vi "Device Under Test Tester.vi"() -> ()   [LabVIEW 2020]
uses:
  <vilib>/Utility/miscctls.llb/LVStringsAndValuesArrayTypeDef_I32.ctl
  <vilib>/Astemes/Triarc Framework/Application/Application.lvclass
  C:/Program Files (x86)/National Instruments/LabVIEW 2020/vi.lib/Astemes/Triarc Framework/Process/Process.lvclass
  Device Under Test/Device Under Test.lvclass
  <vilib>/Astemes/Triarc Framework/View/View.lvclass
  <vilib>/Astemes/Triarc Framework/Process/Process.lvclass/Process.ctl
  <vilib>/Astemes/Triarc Framework/Process/Private/SubVIs/Wait for finish.vi
  <vilib>/Astemes/Triarc Framework/Process/Private/SubVIs/Set Lifecycle State.vi
  <vilib>/Astemes/Triarc Framework/Process/Protected/Messaging/Send Message.vi
  <vilib>/Astemes/Triarc Framework/Process/Private/SubVIs/Handle Debug Data.vi
  <vilib>/Astemes/Triarc Framework/Process/Public/Lifecycle/Get Lifecycle State.vi
  <vilib>/Utility/error.llb/Error Cluster From Error Code.vi
  <vilib>/Astemes/Triarc Framework/Callback/Callback.lvclass
  <vilib>/Astemes/Triarc Framework/Process/Process.lvclass
panel:
  out "timed out?":bool
  in  "Update DUT Status":bool
  out "Self Test Result":bool
  out "Power State":bool
  in  "Self Test":bool
  in  "Power Off":bool
  in  "Power On":bool
  in  "Refresh Modules":bool
  out "Active Modules":string[](array[string])
  in  "Stop Module":bool
  in  "Select Module":i32(ring)=-1 caption="Select Module\nTo send Request to" items=["All"=-1, "DUT 0"=0]
  in  "Run New Module":bool
  in  "Hide Module Panel":bool
  in  "Show Module Panel":bool
  out "Status":string
  # "This VI tests the API for the Module."
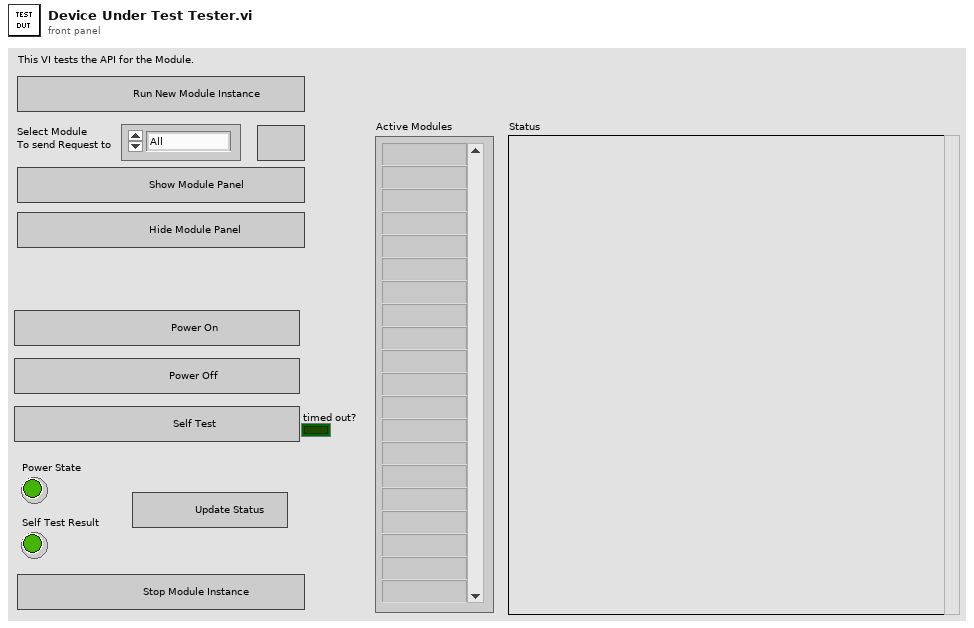
[diagram p1: front panel]
types:
  T1 = typedef "LVStringsAndValuesArrayTypeDef_I32.ctl" = cluster{"String":string, "Value":i32}[]
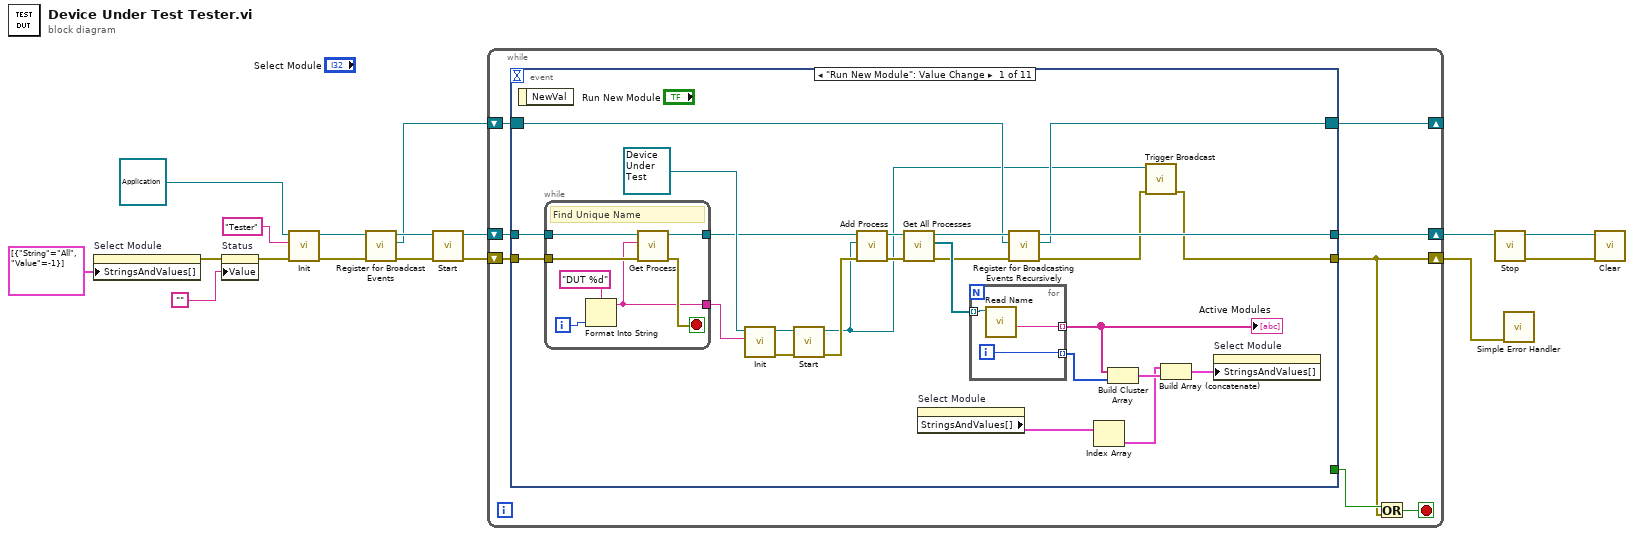
[diagram p0: block diagram]
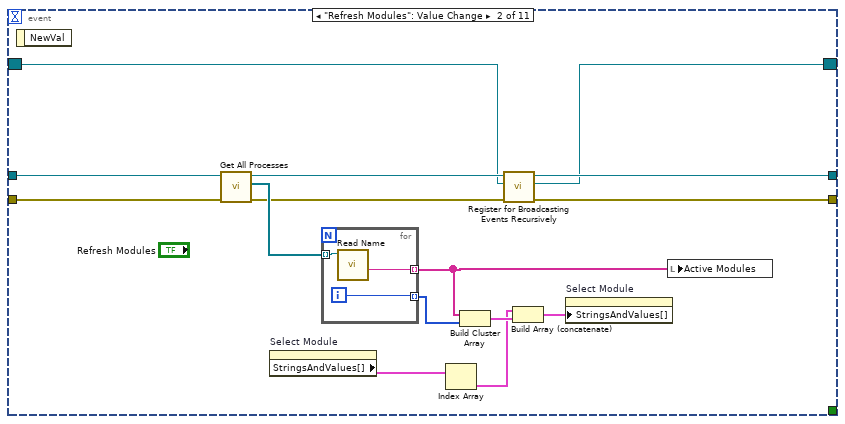
[diagram p2: hidden frame]
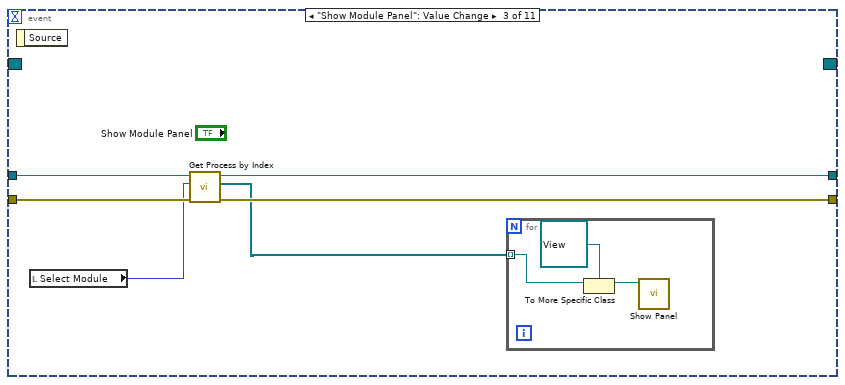
[diagram p3: hidden frame]
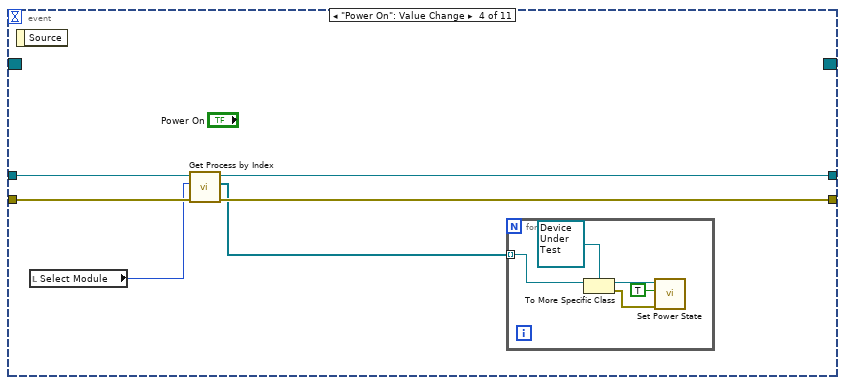
[diagram p4: hidden frame]
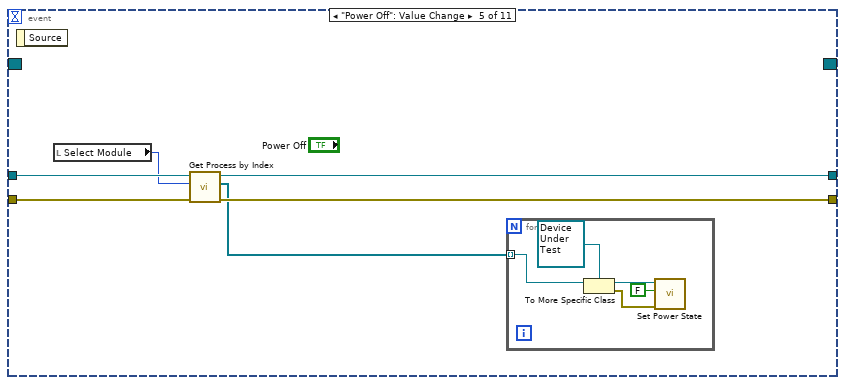
[diagram p5: hidden frame]
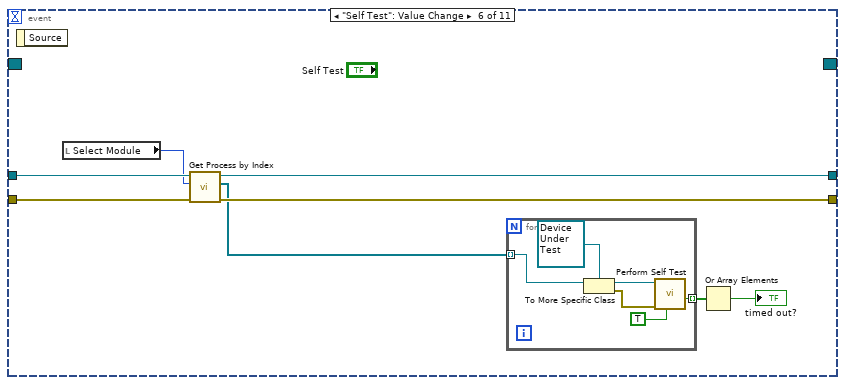
[diagram p6: hidden frame]
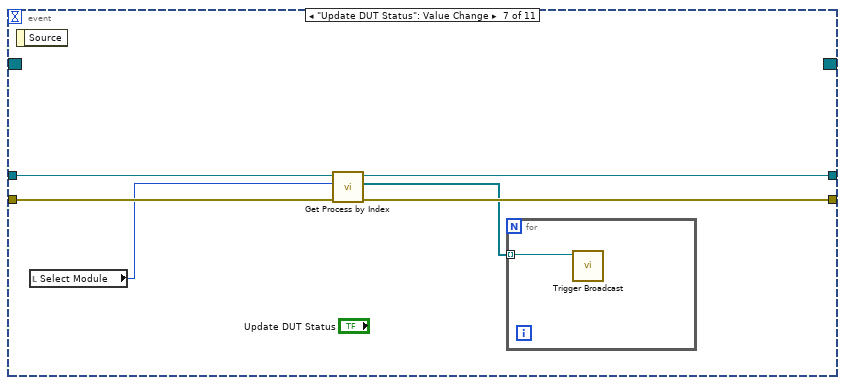
[diagram p7: hidden frame]
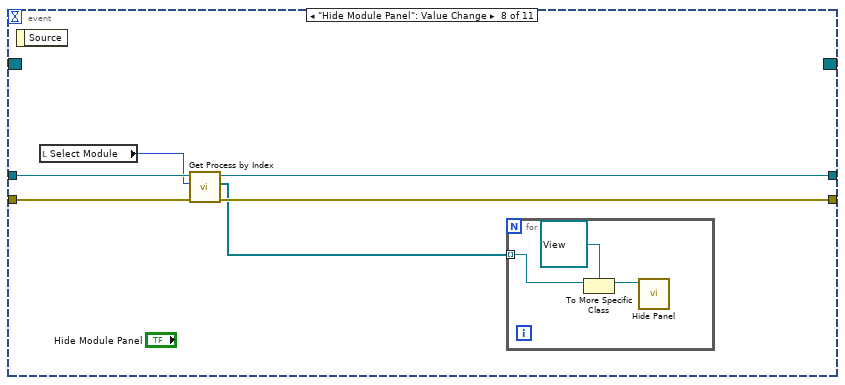
[diagram p8: hidden frame]
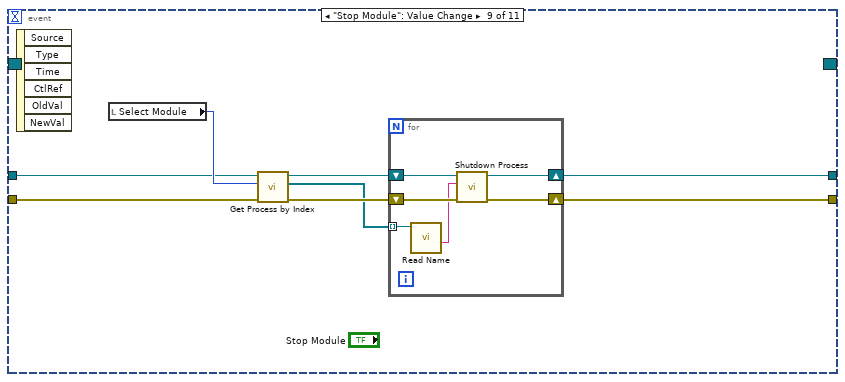
[diagram p9: hidden frame]
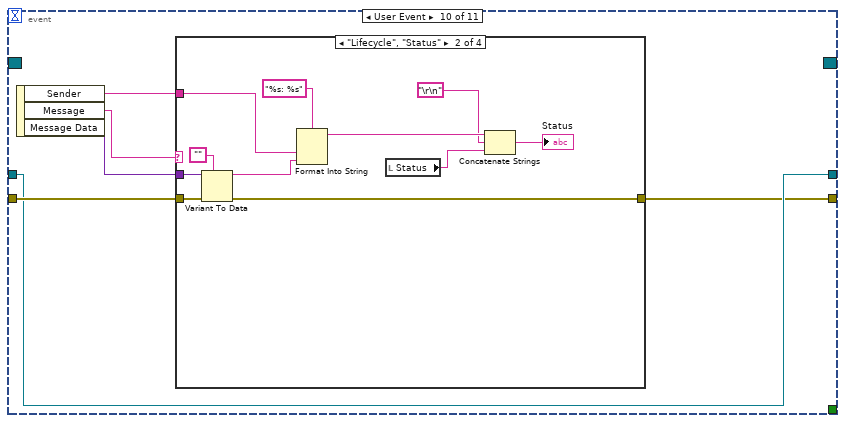
[diagram p10: hidden frame]
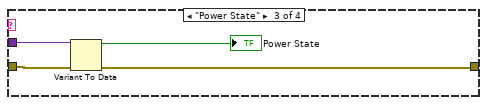
[diagram p12: hidden frame]
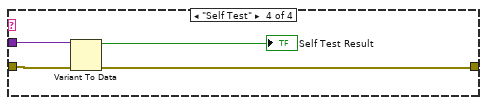
[diagram p13: hidden frame]
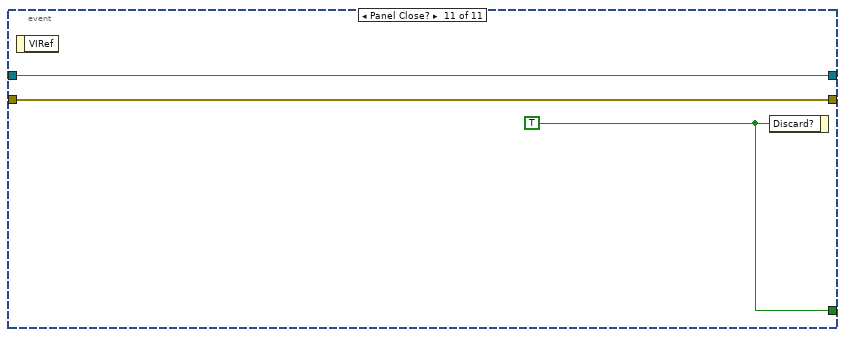
[diagram p14: hidden frame]
diagram:
  n1 = property on="Select Module" class="Ring (strict)"("StringsAndValues[]"=T1 [{"String"="All", "Value"=-1}] ("Strings And Values []")) -> (error out=w3:errorcluster)  [unwired: 2 in, 1 out]
  n2 = property on="Status" class="Str"(error in=w3, "Value"="") -> (error out=w2:errorcluster)  [unwired: 1 in, 1 out]
  n3 = call-dynamic "Init.vi"("error in (no error)"=w2, "Name"="Tester", "Process In"=refnum<class "Application.lvclass"> refnum ("TF.lvlib:Application.lvclass")) -> ("error out"=w4:errorcluster, "Process Out"=w8:refnum<class "Application.lvclass">)  [unwired: 7 in]
  n4 = call <vilib>:"Register for Broadcast Events.vi"("error in (no error)"=w4, "Process In"=w8) -> ("error out"=w6:errorcluster, "Event Registration Refnum Out"=w5:refnum<event-registration>, "Process Out"=w7:refnum<class "Application.lvclass">)  [unwired: 7 in]
  n5 = call <vilib>:"Start.vi"("error in (no error)"=w6, "Process In"=w7) -> ("error out"=w13:errorcluster, "Process Out"=w11:refnum<class "Application.lvclass">)  [unwired: 7 in, 1 out]
  n6 = while {
    shift-right: [w22] -> w17
    shift-left: w13 -> [w25]
    shift-right: [w20] -> w16
    shift-left: w11 -> [w21]
    shift-right: [w18] -> _
    shift-left: w5 -> [w19]
    stop <- w23 stop-if-true
    n7 = event shown="[0] \"Run New Module\": Value Change" {
      selector: w19 -> [w35 w61 _ _ _ _ _ _ _ _ _]
      dyn-events: [w36 w62 _ _ _ _ _ _ _ _ _] -> w18
      timeout: _ -> [_ _ _ _ _ _ _ _ _ _ _]
      tunnel: w25 -> [w32 w70 w84 w93 w104 w117 w129 w136 w145 w158 w181]
      tunnel: [w33 w64 w83 w92 w103 w116 w128 w135 w141 w154 w181] -> w22
      tunnel: [_ _ _ _ _ _ _ _ _ _ w182] -> w24
      tunnel: w21 -> [w31 w69 w82 w91 w102 w115 w127 w134 w146 w156 w180]
      tunnel: [w38 w65 w81 w90 w101 w114 w126 w133 w142 w156 w180] -> w20
      event "Run New Module": Value Change {
        n8 = event-data() -> ()  [unwired: 1 in, 1 out]
        n9 = while {
          tunnel: w32 -> [w56]
          tunnel: w31 -> [w55]
          tunnel: [w54] -> w30
          tunnel: [w51] -> w29
          i -> [w53]
          stop <- w52 stop-if-true
          # "Find Unique Name"
          n10 = Format Into String(format string="DUT %d", w53) -> (resulting string=w51:string)  [unwired: 2 in, 1 out]
          n11 = call <vilib>:"Get Process.vi"("error in (no error)"=w56, "Process Name"=w51, "Application In"=w55) -> ("error out"=w52:errorcluster, "Application Out"=w54:refnum<class "Application.lvclass">)  [unwired: 6 in, 1 out]
        }
        n12 = call-dynamic "Init.vi"("Name"=w29, "View In"=refnum<class "Device Under Test.lvclass"> refnum ("Device Under Test.lvclass")) -> ("error out"=w43:errorcluster, "View Out"=w27:refnum<class "Device Under Test.lvclass">)  [unwired: 8 in]
        n13 = call <vilib>:"Start.vi"("error in (no error)"=w43, "Process In"=w27) -> ("error out"=w28:errorcluster, "Process Out"=w26:refnum<class "Device Under Test.lvclass">)  [unwired: 7 in, 1 out]
        n14 = call <vilib>:"Add Process.vi"("error in (no error)"=w28, "Process"=w26, "Application In"=w30) -> ("error out"=w41:errorcluster, "Application Out"=w42:refnum<class "Application.lvclass">)  [unwired: 7 in]
        n15 = call <vilib>:"Get All Processes.vi"("error in (no error)"=w41, "Application In"=w42) -> ("error out"=w37:errorcluster, "App Processes"=w40:refnum<class "Process.lvclass">[], "Application Out"=w39:refnum<class "Application.lvclass">)  [unwired: 7 in]
        n16 = property on="Select Module" class="Ring (strict)"() -> ("StringsAndValues[]"=w46:T1)  [unwired: 2 in, 2 out]
        n17 = for {
          tunnel: [w58] -> w49 mode=indexing
          tunnel: [w60] -> w48 mode=indexing
          tunnel: w40 -> [w59] mode=indexing
          i -> [w60]
          n18 = call <vilib>:"Read Name.vi"("Process In"=w59) -> ("Name"=w58:string)  [unwired: 7 in, 3 out]
        }
        "Active Modules" <- w49
        n19 = call <vilib>:"Register for Broadcasting Events Recursively.vi"("error in (no error)"=w37, "Event Registration Refnum In"=w35, "Application In"=w39) -> ("error out"=w34:errorcluster, "Event Registration Refnum Out"=w36:refnum<event-registration>, "Application Out"=w38:refnum<class "Application.lvclass">)  [unwired: 6 in]
        n20 = Index Array(array=w46) -> (element=w44:cluster{"String":string, "Value":i32})  [unwired: 1 in]
        n21 = Build Cluster Array(w49, w48) -> (w47:cluster{"Name":string, i32}[])
        n22 = call <vilib>:"Trigger Broadcast.vi"("error in (no error)"=w34, "Process in"=w26) -> ("error out"=w33:errorcluster)  [unwired: 8 in, 1 out]
        n23 = Build Array (concatenate)(w44, w47) -> (w45:cluster{"Name":string, "Value":i32}[])
        n24 = property on="Select Module" class="Ring (strict)"("StringsAndValues[]"=w45) -> ()  [unwired: 2 in, 2 out]
      }
      event "Refresh Modules": Value Change {
        n25 = event-data() -> ()  [unwired: 1 in, 1 out]
        n26 = call <vilib>:"Get All Processes.vi"("error in (no error)"=w70, "Application In"=w69) -> ("error out"=w63:errorcluster, "App Processes"=w68:refnum<class "Process.lvclass">[], "Application Out"=w66:refnum<class "Application.lvclass">)  [unwired: 7 in]
        n27 = property on="Select Module" class="Ring (strict)"() -> ("StringsAndValues[]"=w73:T1)  [unwired: 2 in, 2 out]
        n28 = for {
          tunnel: [w76] -> w67 mode=indexing
          tunnel: [w78] -> w75 mode=indexing
          tunnel: w68 -> [w77] mode=indexing
          i -> [w78]
          n29 = call <vilib>:"Read Name.vi"("Process In"=w77) -> ("Name"=w76:string)  [unwired: 7 in, 3 out]
        }
        n30 = Index Array(array=w73) -> (element=w71:cluster{"String":string, "Value":i32})  [unwired: 1 in]
        n31 = Build Cluster Array(w67, w75) -> (w74:cluster{"Name":string, i32}[])
        n32 = call <vilib>:"Register for Broadcasting Events Recursively.vi"("error in (no error)"=w63, "Event Registration Refnum In"=w61, "Application In"=w66) -> ("error out"=w64:errorcluster, "Event Registration Refnum Out"=w62:refnum<event-registration>, "Application Out"=w65:refnum<class "Application.lvclass">)  [unwired: 6 in]
        n33 = Build Array (concatenate)(w71, w74) -> (w72:cluster{"Name":string, "Value":i32}[])
        n34 = property on="Select Module" class="Ring (strict)"("StringsAndValues[]"=w72) -> ()  [unwired: 2 in, 2 out]
        n35 = local write "Active Modules"(w67) -> ()
      }
      event "Show Module Panel": Value Change {
        n36 = event-data() -> ()  [unwired: 1 in, 1 out]
        n37 = local read "Select Module"() -> (w80:i32)
        n38 = call "Get Process by Index.vi"("error in (no error)"=w84, "Select Module"=w80, "Application in"=w82) -> ("error out"=w83:errorcluster, "Processes"=w79:refnum<class "Process.lvclass">[], "Application out"=w81:refnum<class "Application.lvclass">)  [unwired: 6 in]
        n39 = for {
          tunnel: w79 -> [w87] mode=indexing
          n40 = To More Specific Class(target class=refnum<class "View.lvclass"> refnum ("View In"), reference=w87) -> (specific class reference=w86:refnum<class "View.lvclass">)  [unwired: 1 in, 1 out]
          n41 = call <vilib>:"Show Panel.vi"("View In"=w86) -> ()  [unwired: 9 in, 2 out]
        }
      }
      event "Power On": Value Change {
        n42 = event-data() -> ()  [unwired: 1 in, 1 out]
        n43 = local read "Select Module"() -> (w88:i32)
        n44 = call "Get Process by Index.vi"("error in (no error)"=w93, "Select Module"=w88, "Application in"=w91) -> ("error out"=w92:errorcluster, "Processes"=w89:refnum<class "Process.lvclass">[], "Application out"=w90:refnum<class "Application.lvclass">)  [unwired: 6 in]
        n45 = for {
          tunnel: w89 -> [w98] mode=indexing
          n46 = To More Specific Class(target class=refnum<class "Device Under Test.lvclass"> refnum ("Device Under Test Out"), reference=w98) -> (specific class reference=w97:refnum<class "Device Under Test.lvclass">, error out=w95:errorcluster)  [unwired: 1 in]
          n47 = call "Set Power State.vi"("error in (no error)"=w95, "Power State"=TRUE, "Device Under Test In"=w97) -> ()  [unwired: 7 in, 2 out]
        }
      }
      event "Power Off": Value Change {
        n48 = event-data() -> ()  [unwired: 1 in, 1 out]
        n49 = local read "Select Module"() -> (w99:i32)
        n50 = call "Get Process by Index.vi"("error in (no error)"=w104, "Select Module"=w99, "Application in"=w102) -> ("error out"=w103:errorcluster, "Processes"=w100:refnum<class "Process.lvclass">[], "Application out"=w101:refnum<class "Application.lvclass">)  [unwired: 6 in]
        n51 = for {
          tunnel: w100 -> [w109] mode=indexing
          n52 = To More Specific Class(target class=refnum<class "Device Under Test.lvclass"> refnum ("Device Under Test Out"), reference=w109) -> (specific class reference=w108:refnum<class "Device Under Test.lvclass">, error out=w106:errorcluster)  [unwired: 1 in]
          n53 = call "Set Power State.vi"("error in (no error)"=w106, "Power State"=FALSE, "Device Under Test In"=w108) -> ()  [unwired: 7 in, 2 out]
        }
      }
      event "Self Test": Value Change {
        n54 = event-data() -> ()  [unwired: 1 in, 1 out]
        n55 = local read "Select Module"() -> (w110:i32)
        n56 = call "Get Process by Index.vi"("error in (no error)"=w117, "Select Module"=w110, "Application in"=w115) -> ("error out"=w116:errorcluster, "Processes"=w113:refnum<class "Process.lvclass">[], "Application out"=w114:refnum<class "Application.lvclass">)  [unwired: 6 in]
        n57 = for {
          tunnel: w113 -> [w123] mode=indexing
          tunnel: [w118] -> w112 mode=indexing
          n58 = To More Specific Class(target class=refnum<class "Device Under Test.lvclass"> refnum ("Device Under Test Out"), reference=w123) -> (specific class reference=w122:refnum<class "Device Under Test.lvclass">, error out=w120:errorcluster)  [unwired: 1 in]
          n59 = call "Perform Self Test.vi"("Wait for Reply?"=TRUE, "error in (no error)"=w120, "Device Under Test In"=w122) -> ("Timed out?"=w118:bool)  [unwired: 5 in, 3 out]
        }
        n60 = Or Array Elements(Boolean array=w112) -> (logical OR=→"timed out?":bool)
      }
      event "Update DUT Status": Value Change {
        n61 = event-data() -> ()  [unwired: 1 in, 1 out]
        n62 = local read "Select Module"() -> (w124:i32)
        n63 = call "Get Process by Index.vi"("error in (no error)"=w129, "Select Module"=w124, "Application in"=w127) -> ("error out"=w128:errorcluster, "Processes"=w125:refnum<class "Process.lvclass">[], "Application out"=w126:refnum<class "Application.lvclass">)  [unwired: 6 in]
        n64 = for {
          tunnel: w125 -> [w130] mode=indexing
          n65 = call <vilib>:"Trigger Broadcast.vi"("Process in"=w130) -> ()  [unwired: 9 in, 2 out]
        }
      }
      event "Hide Module Panel": Value Change {
        n66 = event-data() -> ()  [unwired: 1 in, 1 out]
        n67 = local read "Select Module"() -> (w131:i32)
        n68 = call "Get Process by Index.vi"("error in (no error)"=w136, "Select Module"=w131, "Application in"=w134) -> ("error out"=w135:errorcluster, "Processes"=w132:refnum<class "Process.lvclass">[], "Application out"=w133:refnum<class "Application.lvclass">)  [unwired: 6 in]
        n69 = for {
          tunnel: w132 -> [w139] mode=indexing
          n70 = To More Specific Class(target class=refnum<class "View.lvclass"> refnum ("View In"), reference=w139) -> (specific class reference=w138:refnum<class "View.lvclass">)  [unwired: 1 in, 1 out]
          n71 = call <vilib>:"Hide Panel.vi"("View In"=w138) -> ()  [unwired: 9 in, 2 out]
        }
      }
      event "Stop Module": Value Change {
        n72 = event-data() -> ()  [unwired: 1 in, 6 out]
        n73 = local read "Select Module"() -> (w147:i32)
        n74 = call "Get Process by Index.vi"("error in (no error)"=w145, "Select Module"=w147, "Application in"=w146) -> ("error out"=w144:errorcluster, "Processes"=w140:refnum<class "Process.lvclass">[], "Application out"=w143:refnum<class "Application.lvclass">)  [unwired: 6 in]
        n75 = for {
          shift-right: [w150] -> w141
          shift-left: w144 -> [w153]
          shift-right: [w151] -> w142
          shift-left: w143 -> [w152]
          tunnel: w140 -> [w149] mode=indexing
          n76 = call <vilib>:"Read Name.vi"("Process In"=w149) -> ("Name"=w148:string)  [unwired: 7 in, 3 out]
          n77 = call <vilib>:"Shutdown Process.vi"("error in (no error)"=w153, "Process Name"=w148, "Application In"=w152) -> ("error out"=w150:errorcluster, "Application Out"=w151:refnum<class "Application.lvclass">)  [unwired: 7 in]
        }
      }
      event User Event {
        n78 = event-data() -> ("Sender"=w155:string, "Message"=w159:string, "Message Data"=w157:variant)  [unwired: 1 in]
        n79 = case shown="\"Lifecycle\", \"Status\"" w159 {
          tunnel: w158 -> [w160 w171 w174 w178]
          tunnel: w157 -> [_ w170 w175 w179]
          tunnel: w155 -> [_ w168 _ _]
          tunnel: [w160 w165 w172 w177] -> w154
          frame Default {
          }
          frame "Lifecycle", "Status" {
            n80 = Variant To Data(error in=w171, type="", Variant=w170) -> (data=w167:string, error out=w165:errorcluster)
            n81 = Format Into String(format string="%s: %s", w168, w167) -> (resulting string=w162:string)  [unwired: 2 in, 1 out]
            n82 = local read "Status"() -> (w164:string)
            n83 = Concatenate Strings(w162, "\r\n", w164) -> (→"Status":string)
          }
          frame "Power State" {
            n84 = Variant To Data(error in=w174, Variant=w175) -> (data=→"Power State":bool, error out=w172:errorcluster)  [unwired: 1 in]
          }
          frame "Self Test" {
            n85 = Variant To Data(error in=w178, Variant=w179) -> (data=→"Self Test Result":bool, error out=w177:errorcluster)  [unwired: 1 in]
          }
        }
      }
      event Panel Close? {
        w182 = TRUE ("Discard?")
        n86 = event-data() -> ()  [unwired: 1 in, 1 out]
        n87 = event-data("Discard?"=w182) -> ()  [unwired: 1 in, 1 out]
      }
    }
    n88 = Or(x=w24, y=w22) -> (x .or. y?=w23:bool)
  }
  n89 = call <vilib>:"Stop.vi"("Process In"=w16) -> ("error out"=w10:errorcluster, "Process Out"=w9:refnum<class "Application.lvclass">)  [unwired: 8 in, 1 out]
  n90 = call <vilib>:"Simple Error Handler.vi"("error in (no error)"=w17) -> ()  [unwired: 4 in, 5 out]
  n91 = call-dynamic "Clear.vi"("error in (no error)"=w10, "Application In"=w9) -> ()  [unwired: 9 in, 1 out]
